vi "Create Engine Folder and Copy RT Template.vi"(8 "error in":errorcluster, 9 "Project Root":path, 10 "Project Name":string, 11 "CD Template":refnum<class "NIVS_PPL_Inline HW Interface (Inline-Async).lvclass">) -> (0 "error out":errorcluster)   [LabVIEW 2020, in "NIVS_PPL_Inline HW Interface (Inline-Async).lvclass"]
uses:
  NIVS_PPL_Inline HW Interface (Inline-Async).lvclass
  C:/dev/Karthick/FPGA Addons Packages/niveristand-custom-device-wizard/ProjectTemplate/Source/NI VeriStand/Custom Device/Template Classes/NIVS_CD Template/NIVS_CD Template.lvclass
  NIVS_Consolidated_CDW_MetaDataObj/CD Engine lvlib.ctl
  NIVS_Consolidated_CDW_MetaDataObj/Common.ctl
  NIVS_CD Template/NIVS_CD Template.lvclass/NIVS_CD Template.ctl
  NIVS_Consolidated_CDW_MetaDataObj/Common.vi
  NIVS_Consolidated_CDW_MetaDataObj/NIVS_Consolidated_CDW_MetaDataObj.lvclass
  NIVS_CD Template/NIVS_CD Template.lvclass
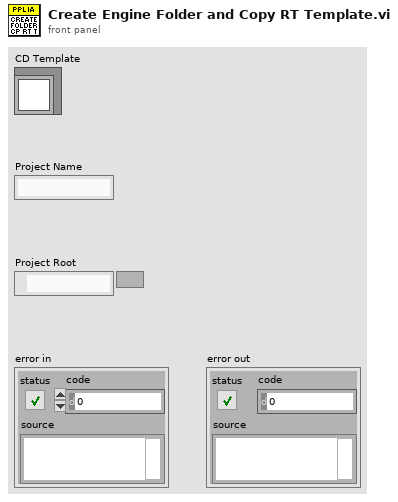
[diagram p1: front panel]
types:
  T1 = typedef "NIVS_Consolidated_CDW_MetaDataObj.lvclass/CD Engine lvlib.ctl" = enum16{"LibraryFileName", "LibraryFolderName", "Engine.FolderName", "Engine.Init.FolderName", "Engine.Run.FolderName", "Engine.Shutdown.FolderName", "Types.FolderName", "Engine.RT Driver VI.TemplatePath", "Engine.RT Driver VI.FileName", "Engine.PPL.RT Driver VI_InlineAsync.FileName", "Engine.RTStateVariables.Name", "Engine.PPL.RTStateVariables.Name", "Engine.RTStateVariables.Name.NoExtension", "Engine.Async.NameExtension", "Engine.Async.TemplateName", "Engine.PPL.Async.TemplateName", "Engine.PPL.Async.InitVSGlobals.Name", "Engine.PPL.RT Driver VI_Inline.FileName", "Engine.LaunchCommandLoop.Name", "Engine.CommandLoop.Name"}
  T2 = typedef "NIVS_Consolidated_CDW_MetaDataObj.lvclass/Common.ctl" = enum16{"ProjectName", "TemplatesFolderName", "PPLTemplatesFolderName", "ProjectTemplatePathAndName", "ProjectPPLTemplatePathAndName", "TimingAndSyncFolderName", "CustomDeviceFolderName", "PathToTemplates", "PathToPPLTemplates", "PathToExplorerPPLTemplates", "PathToEnginePPLTemplates", "PathToConfigurationFile", "ProjectConfigurationName"}
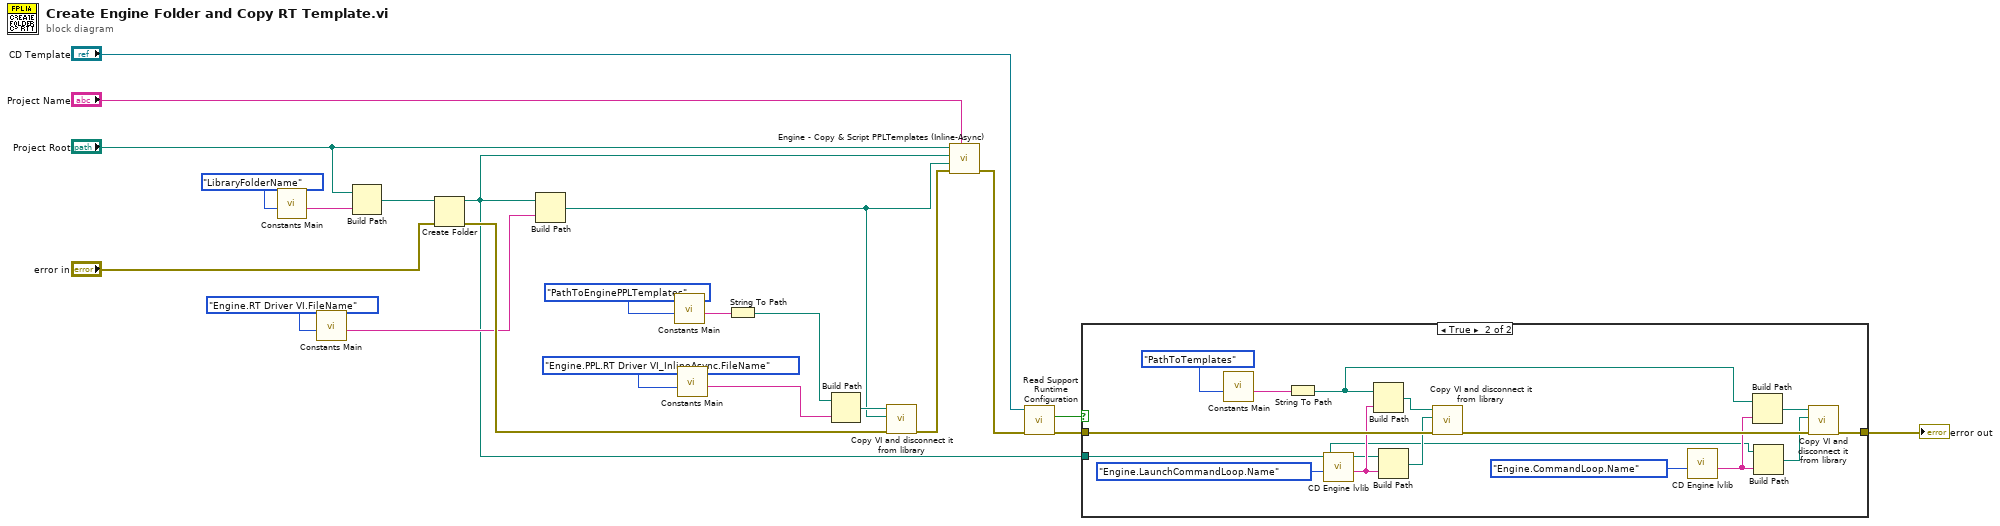
[diagram p0: block diagram]
diagram:
  n1 = call-poly "Constants Main.vi"("Action"=CD_Engine_lvlib."LibraryFolderName") -> ("Output"=w12:string)  [unwired: 10 in]
  n2 = call-poly "Constants Main.vi"("Action"=CD_Engine_lvlib."Engine.RT Driver VI.FileName") -> ("Output"=w16:string)  [unwired: 10 in]
  n3 = Build Path(base path="Project Root", name or relative path=w12) -> (appended path=w2:path)
  n4 = Create Folder(path (use dialog)=w2, error in="error in") -> (created path=w1:path, error out=w23:errorcluster)  [unwired: 1 in, 1 out]
  n5 = Build Path(base path=w1, name or relative path=w16) -> (appended path=w3:path)
  n6 = call-poly "Constants Main.vi"("Action"=Common."PathToEnginePPLTemplates") -> ("Output"=w15:string)  [unwired: 10 in]
  n7 = call-poly "Constants Main.vi"("Action"=CD_Engine_lvlib."Engine.PPL.RT Driver VI_InlineAsync.FileName") -> ("Output"=w7:string)  [unwired: 10 in]
  n8 = String To Path(string=w15) -> (path=w10:path)
  n9 = Build Path(base path=w10, name or relative path=w7) -> (appended path=w14:path)
  n10 = call "Copy VI and disconnect it from library.vi"("error in (no error)"=w23, "VI Target Path"=w3, "VI Source Path"=w14) -> ("error out"=w21:errorcluster)  [unwired: 8 in]
  n11 = call "Engine - Copy & Script PPLTemplates (Inline-Async).vi"("CD Name"="Project Name", "error in (no error)"=w21, "RT Driver VI Path"=w3, "RT Driver Folder Path"=w1, "CD Source Folder Path"="Project Root") -> ("error out"=w19:errorcluster)  [unwired: 6 in]
  n12 = call "Read Support Runtime Configuration.vi"("error in"=w19, "NIVS_CD Template in"="CD Template") -> ("error out"=w20:errorcluster, "Support Runtime Configuration"=w4:bool)  [unwired: 7 in, 1 out]
  n13 = case shown="True" w4 {
    tunnel: [w24 w38] -> w18
    tunnel: w20 -> [w24 w37]
    tunnel: w1 -> [_ w25]
    frame False {
    }
    frame True {
      n14 = call-poly "Constants Main.vi"("Action"=Common."PathToTemplates") -> ("Output"=w32:string)  [unwired: 10 in]
      n15 = String To Path(string=w32) -> (path=w27:path)
      n16 = call "CD Engine lvlib.vi"("Action"=CD_Engine_lvlib."Engine.LaunchCommandLoop.Name") -> ("Output"=w31:string)  [unwired: 10 in]
      n17 = Build Path(base path=w27, name or relative path=w31) -> (appended path=w33:path)
      n18 = Build Path(base path=w25, name or relative path=w31) -> (appended path=w35:path)
      n19 = call "Copy VI and disconnect it from library.vi"("error in (no error)"=w37, "VI Target Path"=w35, "VI Source Path"=w33) -> ("error out"=w39:errorcluster)  [unwired: 8 in]
      n20 = call "CD Engine lvlib.vi"("Action"=CD_Engine_lvlib."Engine.CommandLoop.Name") -> ("Output"=w26:string)  [unwired: 10 in]
      n21 = Build Path(base path=w27, name or relative path=w26) -> (appended path=w28:path)
      n22 = Build Path(base path=w25, name or relative path=w26) -> (appended path=w29:path)
      n23 = call "Copy VI and disconnect it from library.vi"("error in (no error)"=w39, "VI Target Path"=w29, "VI Source Path"=w28) -> ("error out"=w38:errorcluster)  [unwired: 8 in]
    }
  }
  "error out" <- w18
